vi "Test 1.vi"() -> ()   [LabVIEW 2024]
uses:
  DAQmx Actor/Analog Reader/Analog Reader.lvclass
  DAQmx Actor/Digital Writer/Digital Writer.lvclass
  DAQmx Actor/Digital Reader/Digital Reader.lvclass
  <vilib>/ActorFramework/Message Enqueuer/Message Enqueuer.lvclass/Message Enqueuer.ctl
  DAQmx Actor/Digital Writer Messages/Digital Write Single Msg/Digital Write Single Msg.lvclass/Digital Write Single Msg.ctl
  <vilib>/ActorFramework/Message Enqueuer/Enqueue.vi
  <vilib>/ActorFramework/Stop Msg/Stop Msg.lvclass
  DAQmx Actor/Digital Writer Messages/Digital Write Single Msg/Digital Write Single Msg.lvclass
  <vilib>/DAQmx/create/channels.llb/DAQmx Create Channel (AI-Voltage-Basic).vi
  <vilib>/DAQmx/configure/timing.llb/DAQmx Timing (Sample Clock).vi
  <vilib>/DAQmx/create/channels.llb/DAQmx Create Channel (DO-Digital Output).vi
  <vilib>/ActorFramework/Message Priority Queue/Priority Enqueue.vi
  <vilib>/DAQmx/create/channels.llb/DAQmx Create Channel (DI-Digital Input).vi
  <vilib>/ActorFramework/Actor/Actor.lvclass
panel:
  in  "millisecond multiple":u32=10
  out "Waveform Chart":dbl(graph)
  in  "Stop":bool
  out "element":dbl[](array[numeric])
  # "TESTER"
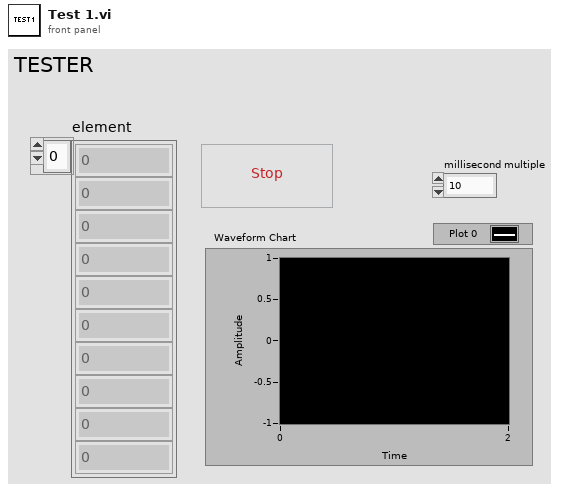
[diagram p1: front panel]
types:
  T1 = cluster{"Actor's Enqueuer":refnum<class "Message Enqueuer.lvclass">, "Actor's Enqueuer":refnum<class "Message Enqueuer.lvclass">, "Actor's Enqueuer":refnum<class "Message Enqueuer.lvclass">}
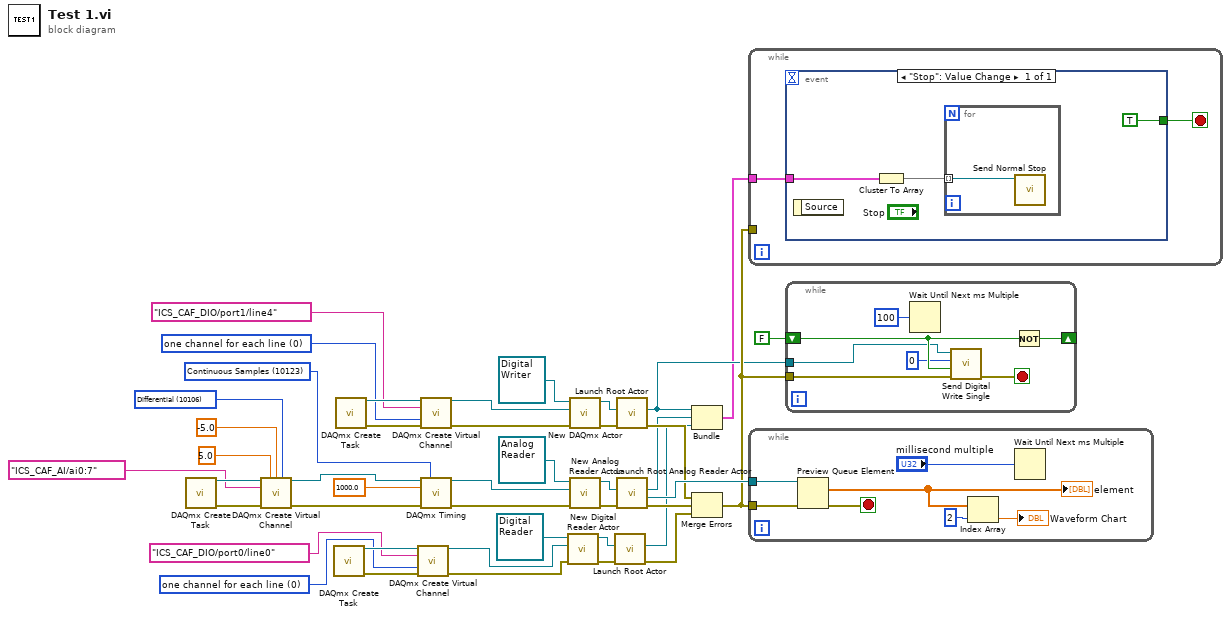
[diagram p0: block diagram]
diagram:
  w5 = 0 items=["one channel for each line", "one channel for all lines"] ("line grouping")
  w25 = 0 items=["one channel for each line", "one channel for all lines"] ("line grouping")
  w35 = 10106 items=["Default"=-1, "RSE"=10083, "NRSE"=10078, "Differential"=10106, "Pseudodifferential"=12529] ("input terminal configuration")
  w38 = 10123 items=["Finite Samples"=10178, "Continuous Samples"=10123, "Hardware Timed Single Point"=12522] ("sample mode")
  n1 = call <vilib>:"DAQmx Create Task.vi"() -> ("task out"=w43:refnum<k21>, "error out"=w41:errorcluster)  [unwired: 14 in]
  n2 = call-poly <vilib>:"DAQmx Create Virtual Channel.vi"("task in"=w43, "maximum value"=5.0, "minimum value"=-5.0, "input terminal configuration"=w35, "physical channels"=tag "ICS_CAF_AI/ai0:7", "error in"=w41) -> ("task out"=w42:refnum<k21>, "error out"=w40:errorcluster)  [unwired: 8 in]
  n3 = call <vilib>:"DAQmx Create Task.vi"() -> ("task out"=w11:refnum<k21>, "error out"=w10:errorcluster)  [unwired: 14 in]
  n4 = call <vilib>:"DAQmx Create Task.vi"() -> ("task out"=w27:refnum<k21>, "error out"=w24:errorcluster)  [unwired: 14 in]
  n5 = call-poly <vilib>:"DAQmx Create Virtual Channel.vi"("task in"=w11, "lines"=tag "ICS_CAF_DIO/port0/line0", "line grouping"=w5, "error in"=w10) -> ("task out"=w9:refnum<k21>, "error out"=w8:errorcluster)  [unwired: 10 in]
  n6 = call-poly <vilib>:"DAQmx Create Virtual Channel.vi"("task in"=w27, "lines"=tag "ICS_CAF_DIO/port1/line4", "line grouping"=w25, "error in"=w24) -> ("task out"=w15:refnum<k21>, "error out"=w22:errorcluster)  [unwired: 10 in]
  n7 = call-poly <vilib>:"DAQmx Timing.vi"("task/channels in"=w42, "sample mode"=w38, "rate"=1000.0, "error in"=w40) -> ("task out"=w30:refnum<k21>, "error out"=w29:errorcluster)  [unwired: 10 in]
  n8 = call-dynamic "New Digital Reader Actor.vi"("error in (no error)"=w8, "DAQmx Task"=w9, "Digital Reader in"=refnum<class "Digital Reader.lvclass"> refnum) -> ("error out"=w12:errorcluster, "Digital Reader out"=w13:refnum<class "Digital Reader.lvclass">)  [unwired: 7 in]
  n9 = call-dynamic "New DAQmx Actor.vi"("error in (no error)"=w22, "DAQmx Task"=w15, "DAQmx Actor in"=refnum<class "Digital Writer.lvclass"> refnum ("DAQmx Actor.lvlib:Digital Writer.lvclass")) -> ("error out"=w20:errorcluster, "DAQmx Actor out"=w21:refnum<class "Digital Writer.lvclass">)  [unwired: 7 in]
  n10 = call-dynamic "New Analog Reader Actor.vi"("error in (no error)"=w29, "DAQmx Task"=w30, "Analog Reader in"=refnum<class "Analog Reader.lvclass"> refnum) -> ("error out"=w28:errorcluster, "Analog Reader out"=w31:refnum<class "Analog Reader.lvclass">)  [unwired: 7 in]
  n11 = call <vilib>:"Launch Root Actor.vi"("error in (no error)"=w12, "Actor"=w13) -> ("error out"=w7:errorcluster, "Actor's Enqueuer"=w2:refnum<class "Message Enqueuer.lvclass">)  [unwired: 8 in]
  n12 = call <vilib>:"Launch Root Actor.vi"("error in (no error)"=w20, "Actor"=w21) -> ("error out"=w19:errorcluster, "Actor's Enqueuer"=w4:refnum<class "Message Enqueuer.lvclass">)  [unwired: 8 in]
  n13 = call "Launch Root Analog Reader Actor.vi"("error in (no error)"=w28, "Analog Reader Actor"=w31) -> ("error out"=w18:errorcluster, "High Speed Data Queue"=w36:refnum<queue>, "Actor's Enqueuer"=w3:refnum<class "Message Enqueuer.lvclass">)  [unwired: 7 in]
  n14 = Bundle("Actor's Enqueuer"=w4, "Actor's Enqueuer"=w3, "Actor's Enqueuer"=w2) -> (w1:T1)  [unwired: 1 in]
  n15 = Merge Errors(w19, w18, w7) -> (w17:errorcluster)
  n16 = while {
    tunnel: w17 -> [_]
    tunnel: w1 -> [w44]
    stop <- w45 stop-if-true
    n17 = event shown="[0] \"Stop\": Value Change" {
      selector: _ -> [_]
      dyn-events: _ -> [_]
      timeout: _ -> [_]
      tunnel: [TRUE] -> w45
      tunnel: w44 -> [w47]
      event "Stop": Value Change {
        n18 = event-data() -> ()  [unwired: 1 in, 1 out]
        n19 = Cluster To Array(cluster=w47) -> (array=w46:refnum<class "Message Enqueuer.lvclass">[])
        n20 = for {
          tunnel: w46 -> [w49] mode=indexing
          n21 = call <vilib>:"Send Normal Stop.vi"("Message Enqueuer"=w49) -> ()  [unwired: 10 in, 1 out]
        }
      }
    }
  }
  n22 = while {
    tunnel: w36 -> [w56]
    tunnel: w17 -> [w53]
    stop <- w55 stop-if-true
    n23 = Preview Queue Element(queue=w56, error in (no error)=w53) -> (element=w52:dbl[], error out=w55:errorcluster)  [unwired: 1 in, 2 out]
    "element" <- w52
    n24 = Index Array(array=w52, index=2) -> (element=→"Waveform Chart":dbl)
    n25 = Wait Until Next ms Multiple(millisecond multiple="millisecond multiple") -> ()  [unwired: 1 out]
  }
  n26 = while {
    tunnel: w4 -> [w60]
    tunnel: w17 -> [w59]
    shift-right: [w63] -> _
    shift-left: FALSE -> [w61]
    stop <- w58 stop-if-true
    n27 = Wait Until Next ms Multiple(millisecond multiple=u32 100) -> ()  [unwired: 1 out]
    n28 = call "Send Digital Write Single.vi"("error in (no error)"=w59, "Digital Data"=w61, "Channel Index"=0, "Message Enqueuer"=w60) -> ("error out"=w58:errorcluster)  [unwired: 6 in, 1 out]
    n29 = Not(x=w61) -> (.not. x?=w63:bool)
  }
